vi "Warning Dialog.vi"(11 "Path":path) -> (3 "Continue?":bool)   [LabVIEW 2019, in "Panther Dashboard.lvlib"]
uses:
  Panther Dashboard.lvlib
panel:
  in  "Cancel":bool
  in  "Continue":bool
  out "Message":string
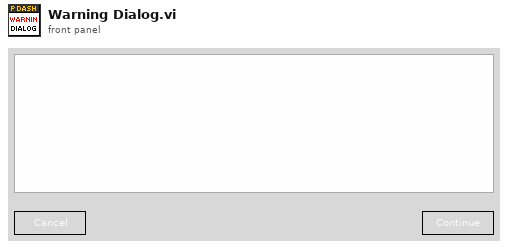
[diagram p1: front panel]
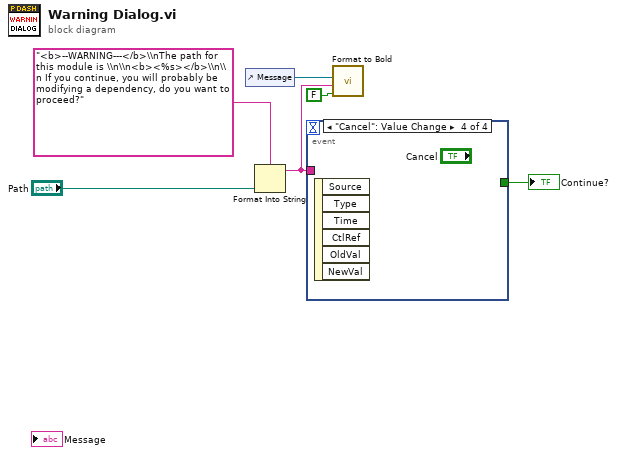
[diagram p0: block diagram]
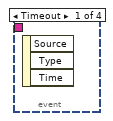
[diagram p2: hidden frame]
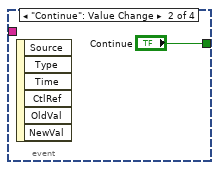
[diagram p3: hidden frame]
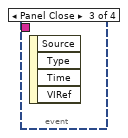
[diagram p4: hidden frame]
diagram:
  n1 = control-ref of="Message"() -> (w5:refnum<vi>)
  n2 = Format Into String(format string="<b>--WARNING---</b>\\nThe path for this module is \\n\\n<b><%s></b>\\n\\n If you continue, you will probably be modifying a dependency, do you want to proceed?" ("message"), "Path") -> (resulting string=w1:string)  [unwired: 2 in, 1 out]
  n3 = event shown="[3] \"Cancel\": Value Change" {
    selector: _ -> [_ _ _ _]
    dyn-events: _ -> [_ _ _ _]
    timeout: _ -> [_ _ _ _]
    tunnel: [_ "Continue" _ _] -> w2
    tunnel: w1 -> [_ _ _ _]
    event Timeout {
      n4 = event-data() -> ()  [unwired: 1 in, 3 out]
    }
    event "Continue": Value Change {
      n5 = event-data() -> ()  [unwired: 1 in, 6 out]
    }
    event Panel Close {
      n6 = event-data() -> ()  [unwired: 1 in, 4 out]
    }
    event "Cancel": Value Change {
      n7 = event-data() -> ()  [unwired: 1 in, 6 out]
    }
  }
  "Continue?" <- w2
  n8 = call "Format to Bold.vi"("Adjust Height?"=FALSE, "String Value"=w1, "String Ref"=w5) -> ()  [unwired: 9 in]
